vi "Configure Channel Linkage.vi"(8 "error in (no error)":errorcluster, 9 "Channel 2":T1, 10 "Channel 1":T1, 11 "DG645 in":refnum<class "DG645.lvclass">) -> (0 "error out":errorcluster, 3 "DG645 out":refnum<class "DG645.lvclass">)   [LabVIEW 2018, in "DG645.lvlib" / "DG645.lvclass"]
uses:
  DG645.lvclass
  PPLs/Digital Delay Generator/Parent/Digital Delay Generator.lvlibp/Custom Controls/Channel.ctl
  DG645.lvclass/DG645.ctl
  <instrlib>/Stanford Research DG645/Stanford Research DG645.lvlib
  PPLs/Digital Delay Generator/Parent/Digital Delay Generator.lvlibp/Digital Delay Generator.lvclass
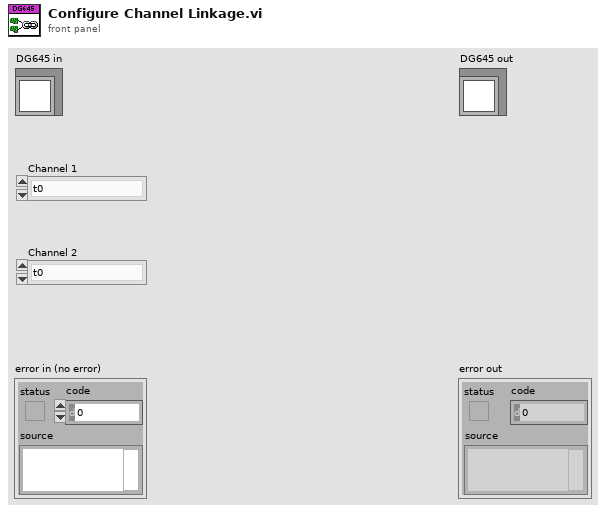
[diagram p1: front panel]
types:
  T1 = typedef "Digital Delay Generator.lvlibp/Digital Delay Generator.lvclass/Channel.ctl" = enum16{"t0", "A", "B", "C", "D", "E", "F", "G", "H"}
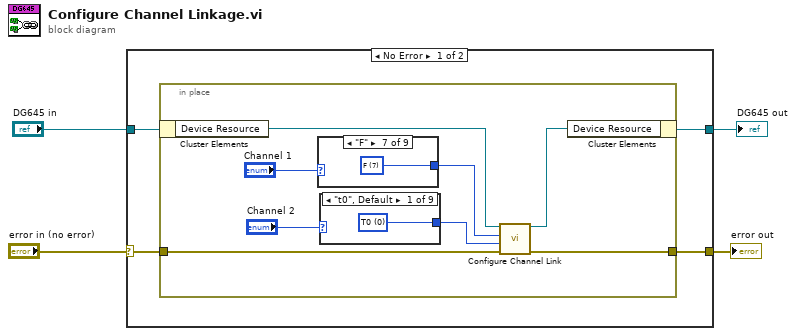
[diagram p0: block diagram]
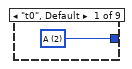
[diagram p2: hidden frame]
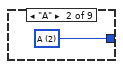
[diagram p3: hidden frame]
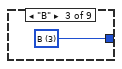
[diagram p4: hidden frame]
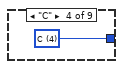
[diagram p5: hidden frame]
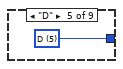
[diagram p6: hidden frame]
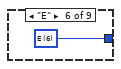
[diagram p7: hidden frame]
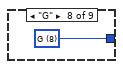
[diagram p8: hidden frame]
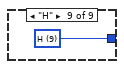
[diagram p9: hidden frame]
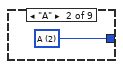
[diagram p10: hidden frame]
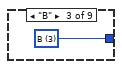
[diagram p11: hidden frame]
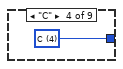
[diagram p12: hidden frame]
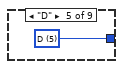
[diagram p13: hidden frame]
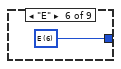
[diagram p14: hidden frame]
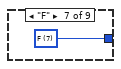
[diagram p15: hidden frame]
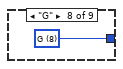
[diagram p16: hidden frame]
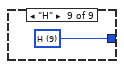
[diagram p17: hidden frame]
diagram:
  n1 = case shown="No Error" "error in (no error)" {
    selector: "error in (no error)" -> [w7 w35]
    tunnel: "DG645 in" -> [w8 w36]
    tunnel: [w5 w36] -> w2
    tunnel: [w6 w35] -> w1
    frame No Error {
      n2 = in-place {
        in-place-border: w7 -> [w16]
        in-place-border: [w15] -> w6
        n3 = in-place-cluster #1(w8) -> ("Device Resource"=w14:refnum<visa-resource-name>)
        n4 = case shown="\"F\"" "Channel 1" {
          tunnel: [w17 w18 w19 w20 w21 w22 w23 w24 w25] -> w10
          frame "t0", Default {
            w17 = u16 2 items=["T0"=0, "A"=2, "B"=3, "C"=4, "D"=5, "E"=6, "F"=7, "G"=8, "H"=9] ("Reference Channel (0:T0)")
          }
          frame "A" {
            w18 = u16 2 items=["T0"=0, "A"=2, "B"=3, "C"=4, "D"=5, "E"=6, "F"=7, "G"=8, "H"=9] ("Reference Channel (0:T0)")
          }
          frame "B" {
            w19 = u16 3 items=["T0"=0, "A"=2, "B"=3, "C"=4, "D"=5, "E"=6, "F"=7, "G"=8, "H"=9] ("Reference Channel (0:T0)")
          }
          frame "C" {
            w20 = u16 4 items=["T0"=0, "A"=2, "B"=3, "C"=4, "D"=5, "E"=6, "F"=7, "G"=8, "H"=9] ("Reference Channel (0:T0)")
          }
          frame "D" {
            w21 = u16 5 items=["T0"=0, "A"=2, "B"=3, "C"=4, "D"=5, "E"=6, "F"=7, "G"=8, "H"=9] ("Reference Channel (0:T0)")
          }
          frame "E" {
            w22 = u16 6 items=["T0"=0, "A"=2, "B"=3, "C"=4, "D"=5, "E"=6, "F"=7, "G"=8, "H"=9] ("Reference Channel (0:T0)")
          }
          frame "F" {
            w23 = u16 7 items=["T0"=0, "A"=2, "B"=3, "C"=4, "D"=5, "E"=6, "F"=7, "G"=8, "H"=9] ("Reference Channel (0:T0)")
          }
          frame "G" {
            w24 = u16 8 items=["T0"=0, "A"=2, "B"=3, "C"=4, "D"=5, "E"=6, "F"=7, "G"=8, "H"=9] ("Reference Channel (0:T0)")
          }
          frame "H" {
            w25 = u16 9 items=["T0"=0, "A"=2, "B"=3, "C"=4, "D"=5, "E"=6, "F"=7, "G"=8, "H"=9] ("Reference Channel (0:T0)")
          }
        }
        n5 = case shown="\"t0\", Default" "Channel 2" {
          tunnel: [w26 w27 w28 w29 w30 w31 w32 w33 w34] -> w9
          frame "t0", Default {
            w26 = u16 0 items=["T0"=0, "A"=2, "B"=3, "C"=4, "D"=5, "E"=6, "F"=7, "G"=8, "H"=9] ("Reference Channel (0:T0)")
          }
          frame "A" {
            w27 = u16 2 items=["T0"=0, "A"=2, "B"=3, "C"=4, "D"=5, "E"=6, "F"=7, "G"=8, "H"=9] ("Reference Channel (0:T0)")
          }
          frame "B" {
            w28 = u16 3 items=["T0"=0, "A"=2, "B"=3, "C"=4, "D"=5, "E"=6, "F"=7, "G"=8, "H"=9] ("Reference Channel (0:T0)")
          }
          frame "C" {
            w29 = u16 4 items=["T0"=0, "A"=2, "B"=3, "C"=4, "D"=5, "E"=6, "F"=7, "G"=8, "H"=9] ("Reference Channel (0:T0)")
          }
          frame "D" {
            w30 = u16 5 items=["T0"=0, "A"=2, "B"=3, "C"=4, "D"=5, "E"=6, "F"=7, "G"=8, "H"=9] ("Reference Channel (0:T0)")
          }
          frame "E" {
            w31 = u16 6 items=["T0"=0, "A"=2, "B"=3, "C"=4, "D"=5, "E"=6, "F"=7, "G"=8, "H"=9] ("Reference Channel (0:T0)")
          }
          frame "F" {
            w32 = u16 7 items=["T0"=0, "A"=2, "B"=3, "C"=4, "D"=5, "E"=6, "F"=7, "G"=8, "H"=9] ("Reference Channel (0:T0)")
          }
          frame "G" {
            w33 = u16 8 items=["T0"=0, "A"=2, "B"=3, "C"=4, "D"=5, "E"=6, "F"=7, "G"=8, "H"=9] ("Reference Channel (0:T0)")
          }
          frame "H" {
            w34 = u16 9 items=["T0"=0, "A"=2, "B"=3, "C"=4, "D"=5, "E"=6, "F"=7, "G"=8, "H"=9] ("Reference Channel (0:T0)")
          }
        }
        n6 = call <instrlib>:"Configure Channel Link.vi"("VISA resource name"=w14, "Channel To Modify (2:A)"=w10, "Reference Channel (0:T0)"=w9, "error in (no error)"=w16) -> ("VISA resource name out"=w13:refnum<visa-resource-name>, "error out"=w15:errorcluster)  [unwired: 10 in]
        n7 = in-place-cluster #1("Device Resource"=w13) -> (w5:refnum<class "DG645.lvclass">)
      }
    }
    frame Error {
    }
  }
  "error out" <- w1
  "DG645 out" <- w2
